vi "Store Targetting Output.vi"(10 "mode":T1(ring), 11 "Targetting Input":T3) -> (3 "Targetting Output":T3)   [LabVIEW 2011]
uses:
  Camera State.ctl
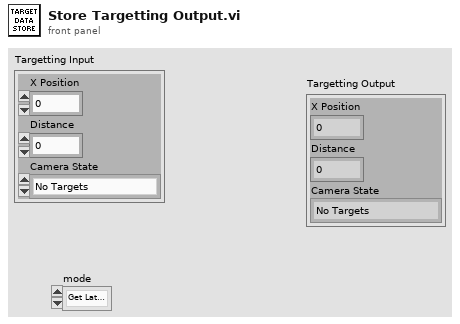
[diagram p1: front panel]
types:
  T1 = enum16{"Get Latest Data", "Get Local Data", "Get Remote Data", "Set Local Data", "Set Remote Data"}
  T2 = typedef "Camera State.ctl" = enum16{"No Targets", "Low Confidence", "Medium Confidence", "High Confidence", "Camera Error"}
  T3 = cluster{"X Position":dbl, "Distance":dbl, "Camera State":T2}
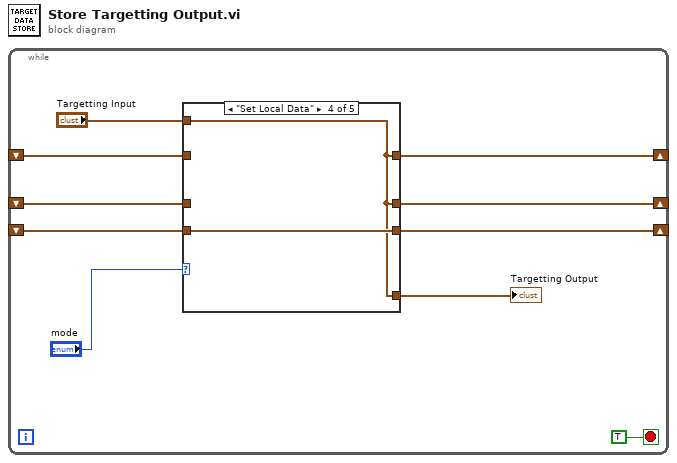
[diagram p0: block diagram]
diagram:
  n1 = while {
    shift-right: [w3] -> _
    shift-left: _ -> [w2]
    shift-right: [w7] -> _
    shift-left: _ -> [w8]
    shift-right: [w4] -> _
    shift-left: _ -> [w5]
    stop <- TRUE stop-if-true
    n2 = case shown="\"Set Local Data\"" "mode" {
      tunnel: w8 -> [w12 w16 w18 _ w23]
      tunnel: [w12 w16 w18 w20 w23] -> w7
      tunnel: [w13 w16 w19 w20 w22] -> w6
      tunnel: w5 -> [w11 w14 w19 w21 _]
      tunnel: [w11 w14 w19 w21 w22] -> w4
      tunnel: [w13 w15 w17 w20 w22] -> w3
      tunnel: w2 -> [w13 w15 w17 _ _]
      tunnel: "Targetting Input" -> [_ _ _ w20 w22]
      frame "Get Latest Data", Default {
      }
      frame "Get Local Data" {
      }
      frame "Get Remote Data" {
      }
      frame "Set Local Data" {
      }
      frame "Set Remote Data" {
      }
    }
    "Targetting Output" <- w6
  }
